vi "sendValue.vi"(8 "error in (no error)":errorcluster, 10 "data":variant, 11 "start in":refnum<class "start.lvclass">) -> (0 "error out":errorcluster, 2 "function return":i32, 3 "start out":refnum<class "start.lvclass">)   [LabVIEW 2016, in "SALLV_MtAtElectrometer_Messaging.lvlib" / "start.lvclass"]
uses:
  start.lvclass
  ts_sallv_MtAtElectrometer/DataTypes/command_start.ctl
  start.lvclass/start.ctl
  ts_sallv_MtAtElectrometer/SALLV_MtAtElectrometer.lvlib
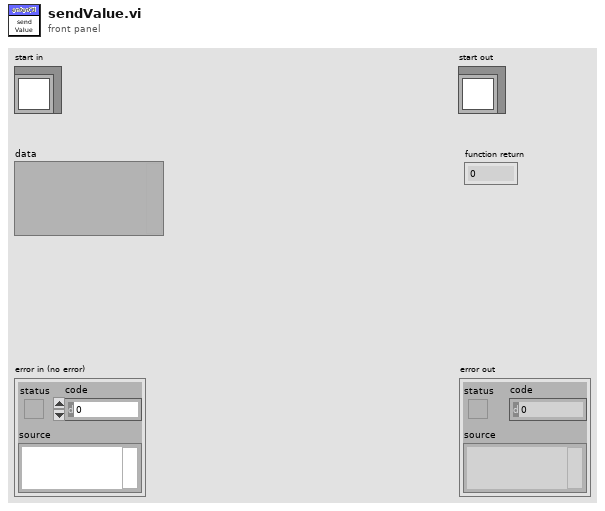
[diagram p1: front panel]
types:
  T1 = typedef "SALLV_MtAtElectrometer.lvlib/command_start.ctl" = cluster{"settingsToApply":string}
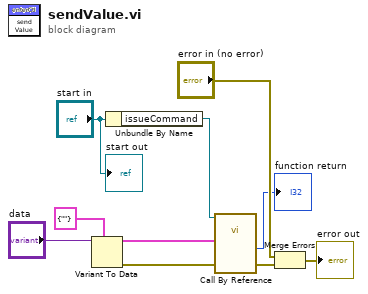
[diagram p0: block diagram]
diagram:
  n1 = Variant To Data(type=T1 {"settingsToApply"=""} ("command_start"), Variant="data") -> (data=w2:T1, error out=w3:errorcluster)  [unwired: 1 in]
  n2 = Unbundle By Name("start in") -> ("issueCommand"=w8:refnum<vi>)
  n3 = call-by-ref "?"(reference=w8, "error in (no error)"=w3, "command_start_Ctl"=w2) -> ("error out"=w9:errorcluster, "function return"=→"function return":i32)  [unwired: 8 in, 3 out]
  n4 = Merge Errors("error in (no error)", w9) -> (→"error out":errorcluster)
  "start out" <- "start in"
